vi "StartHeadingTest.vi"(9 "Target POS":dbl[](array[numeric])=[1.63875, 0.805, -1.5708], 11 "Start POS":dbl[](array[numeric])=[1.3859, 1.2768, -2.8198]) -> (1 "Heading rad back":dbl, 3 "Heading rad":dbl, 5 "InRange":bool)   [LabVIEW 2018]
panel:
  out "Out deg":dbl
  out "In deg":dbl
  out "included deg":dbl
  out "Target deg":dbl
  out "Target theta":dbl
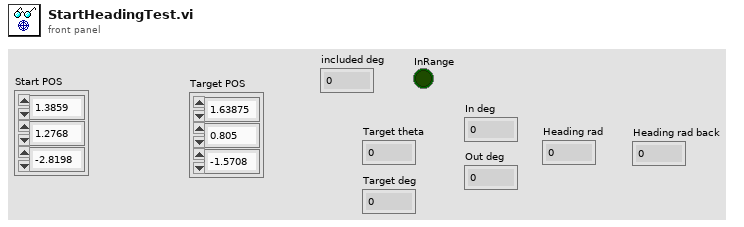
[diagram p1: front panel]
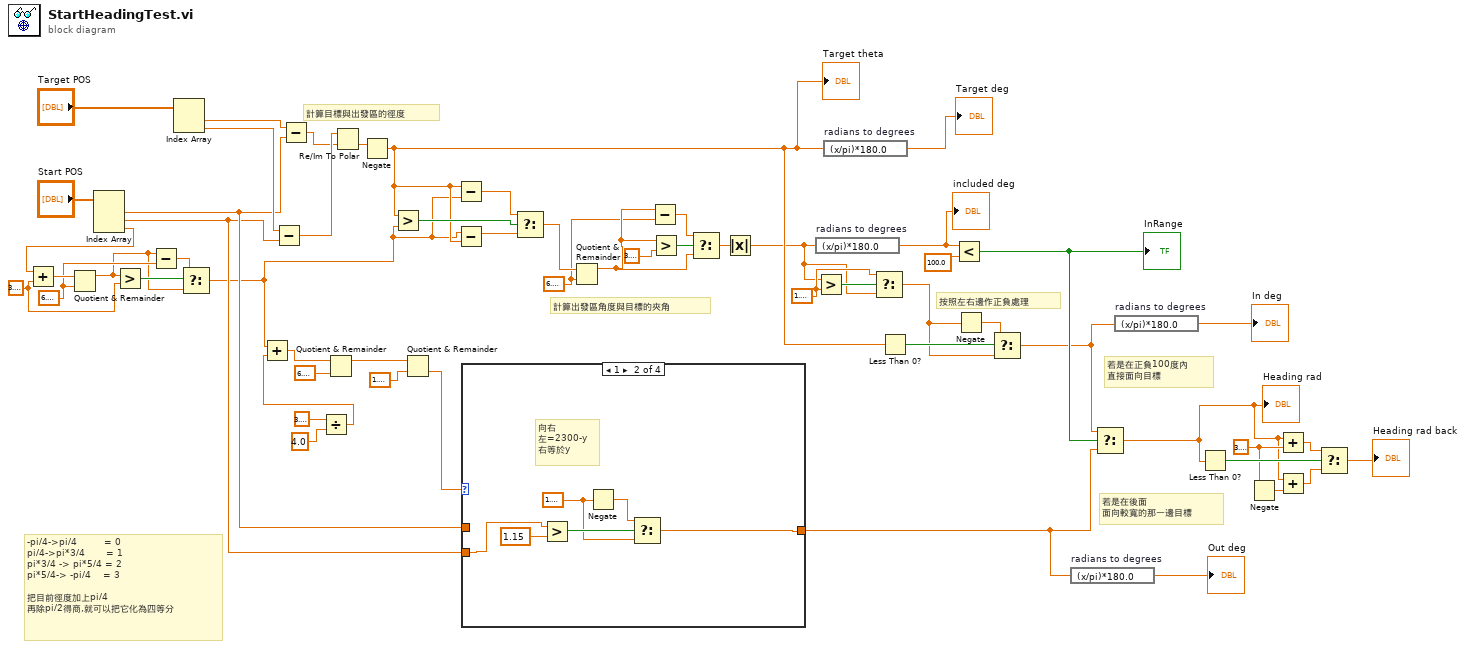
[diagram p0: block diagram]
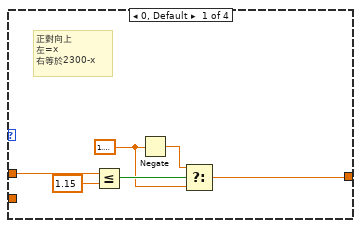
[diagram p2: hidden frame]
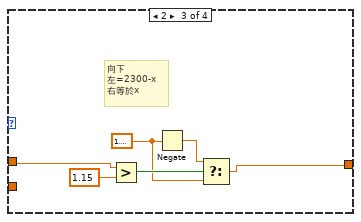
[diagram p3: hidden frame]
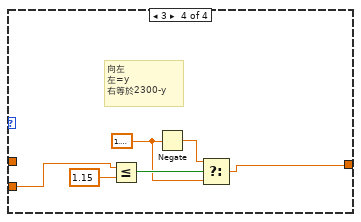
[diagram p4: hidden frame]
diagram:
  w3 = 6.283185307179586
  w6 = 3.141592653589793
  w11 = 3.141592653589793
  w25 = 1.5707963267948966
  w40 = 6.283185307179586
  # "若是在後面\n面向較寬的那一邊目標"
  # "若是在正負100度內\n直接面向目標"
  # "按照左右邊作正負處理"
  # "-pi/4->pi/4         = 0\npi/4->pi*3/4       = 1\npi*3/4 -> pi*5/4 = 2\npi*5/4-> -pi/4    = 3\n\n把目前徑度加上pi/4\n再除pi/2得商,就可以把它化為四等分"
  # "計算出發區角度與目標的夾角"
  # "計算目標與出發區的徑度"
  n1 = Index Array(array="Start POS") -> (element #1=w30:dbl, element #2=w29:dbl, element #3=w8:dbl)  [unwired: 3 in]
  n2 = Add(x=w8, y=w6) -> (x+y=w7:dbl)
  n3 = Quotient & Remainder(x=w7, y=w3) -> (x-y*floor(x/y)=w2:dbl)  [unwired: 1 out]
  n4 = Greater?(x=w2, y=w6) -> (0:w5:bool)
  n5 = Subtract(x=w2, y=w3) -> (x-y=w4:dbl)
  n6 = Index Array(array="Target POS") -> (element #1=w55:dbl, element #2=w54:dbl)  [unwired: 2 in]
  n7 = Select(t=w4, s=w5, f=w2) -> (s? t:f=w1:dbl)
  n8 = Subtract(x=w54, y=w29) -> (x-y=w52:dbl)
  n9 = Subtract(x=w55, y=w30) -> (x-y=w51:dbl)
  n10 = Divide(x=3.141592653589793, y=4.0) -> (x/y=w33:dbl)
  n11 = Add(x=w1, y=w33) -> (x+y=w34:dbl)
  n12 = Quotient & Remainder(x=w34, y=6.283185307179586) -> (x-y*floor(x/y)=w37:dbl)  [unwired: 1 out]
  n13 = Re/Im To Polar(2:w51, 3:w52) -> (0:w50:dbl)  [unwired: 1 out]
  n14 = Negate(x=w50) -> (-x=w24:dbl)
  "Target theta" <- w24
  n15 = Greater?(x=w24, y=w1) -> (0:w42:bool)
  n16 = Quotient & Remainder(x=w37, y=1.5707963267948966) -> (floor(x/y)=w31:dbl)  [unwired: 1 out]
  n17 = Subtract(x=w24, y=w1) -> (x-y=w44:dbl)
  n18 = Subtract(x=w1, y=w24) -> (x-y=w43:dbl)
  n19 = case shown="1" w31 {
    tunnel: w30 -> [w63 _ w71 _]
    tunnel: w29 -> [_ w65 _ w77]
    tunnel: [w58 w64 w70 w76] -> w16
    frame 0, Default {
      w59 = 1.5707963267948966
      # "正對向上\n左=x\n右等於2300-x"
      n20 = Less Or Equal?(x=w63, y=1.15) -> (x <= y?=w61:bool)
      n21 = Negate(x=w59) -> (-x=w60:dbl)
      n22 = Select(t=w60, s=w61, f=w59) -> (s? t:f=w58:dbl)
    }
    frame 1 {
      w66 = 1.5707963267948966
      # "向右\n左=2300-y\n右等於y"
      n23 = Greater?(x=w65, y=1.15) -> (0:w68:bool)
      n24 = Negate(x=w66) -> (-x=w67:dbl)
      n25 = Select(t=w67, s=w68, f=w66) -> (s? t:f=w64:dbl)
    }
    frame 2 {
      w72 = 1.5707963267948966
      # "向下\n左=2300-x\n右等於x"
      n26 = Greater?(x=w71, y=1.15) -> (0:w74:bool)
      n27 = Negate(x=w72) -> (-x=w73:dbl)
      n28 = Select(t=w73, s=w74, f=w72) -> (s? t:f=w70:dbl)
    }
    frame 3 {
      w78 = 1.5707963267948966
      # "向左\n左=y\n右等於2300-y"
      n29 = Less Or Equal?(x=w77, y=1.15) -> (x <= y?=w80:bool)
      n30 = Negate(x=w78) -> (-x=w79:dbl)
      n31 = Select(t=w79, s=w80, f=w78) -> (s? t:f=w76:dbl)
    }
  }
  n32 = Select(t=w44, s=w42, f=w43) -> (s? t:f=w41:dbl)
  n33 = Quotient & Remainder(x=w41, y=w40) -> (x-y*floor(x/y)=w45:dbl)  [unwired: 1 out]
  n34 = Subtract(x=w45, y=w40) -> (x-y=w47:dbl)
  n35 = Greater?(x=w45, y=3.141592653589793) -> (0:w48:bool)
  n36 = Select(t=w47, s=w48, f=w45) -> (s? t:f=w39:dbl)
  n37 = Absolute Value(x=w39) -> (abs(x)=w23:dbl)
  n38 = expression code="(x/pi)*180.0" "radians to degrees"(w23) -> (w27:dbl)
  "included deg" <- w27
  n39 = Greater?(x=w23, y=w25) -> (0:w26:bool)
  n40 = expression code="(x/pi)*180.0" "radians to degrees"(w24) -> (→"Target deg":dbl)
  n41 = Select(t=w25, s=w26, f=w23) -> (s? t:f=w21:dbl)
  n42 = Less Than 0?(x=w24) -> (x < 0?=w22:bool)
  n43 = Less?(x=w27, y=100.0) -> (x < y?=w20:bool)
  "InRange" <- w20
  n44 = Negate(x=w21) -> (-x=w28:dbl)
  n45 = Select(t=w28, s=w22, f=w21) -> (s? t:f=w19:dbl)
  n46 = expression code="(x/pi)*180.0" "radians to degrees"(w16) -> (→"Out deg":dbl)
  n47 = Select(t=w19, s=w20, f=w16) -> (s? t:f=w10:dbl)
  "Heading rad" <- w10
  n48 = expression code="(x/pi)*180.0" "radians to degrees"(w19) -> (→"In deg":dbl)
  n49 = Less Than 0?(x=w10) -> (x < 0?=w15:bool)
  n50 = Negate(x=w11) -> (-x=w12:dbl)
  n51 = Add(x=w10, y=w11) -> (x+y=w14:dbl)
  n52 = Add(x=w10, y=w12) -> (x+y=w13:dbl)
  n53 = Select(t=w14, s=w15, f=w13) -> (s? t:f=→"Heading rad back":dbl)
